vi "myRIO-1900 Customized FPGA.vi"() -> ()   [LabVIEW 2013]
doc: "This VI contains the NI myRIO FPGA shipping personality. This VI compiles and runs on the NI myRIO FPGA target. You can modify this VI to suit your application needs. National Instruments recommends that you only add new FPGA code to this VI and do not modify the existing code. This VI might not work correctly with the myRIO VIs if you modify the existing code."
uses:
  Sub VIs/Utilities/Start Boolean.ctl
  <vilib>/Platform/TimedLoop/XDataNode/timing_clust.ctl
  <vilib>/Platform/TimedLoop/XDataNode/nitl_modes.ctl
  <vilib>/Platform/TimedLoop/XDataNode/wakeup.ctl
  <vilib>/rvi/Emulation/niFpgaSctlEmulationGetInTimedLoop.vi
  <vilib>/rvi/Emulation/niFpgaEmulationReportErrorSimple.vi
  <vilib>/rvi/Emulation/niFpgaGetClockAttributes.vi
  <vilib>/rvi/Emulation/niFpgaCriticalErrorInLSC.vi
  <vilib>/rvi/interface/RandomDataEmulation/niFpgaRandomDataHandleErrors.vi
  <vilib>/rvi/interface/RandomDataEmulation/nirviRandomDataFPGAFIFO.vi
  <vilib>/rvi/eio/common/nirviEmuTemplateMethod_errors.vi
  <vilib>/rvi/eio/common/nirviEmuTemplatePropertyGet_noerrors.vi
  <vilib>/Platform/TimedLoop/XDataNode/XDataNode.xnode
  <vilib>/rvi/DataTransferAndStorage/Container/XNode/niFpgaContainer.xnode
  <vilib>/rvi/interface/RandomDataEmulation/nirviRandomDataFpgaReadWriteTemplate.vi
  <vilib>/eio/EIONode/EIONode.xnode
  <vilib>/eio/EIOPropertyNode/EIOPropertyNode.xnode
  <vilib>/Platform/TimedLoop/XDataNode/XDNodeRunTimeDep.lvlib
  <vilib>/rvi/eio/common/nirviEmuTemplatePropertyGet_errors.vi
  <vilib>/rvi/eio/common/nirviEmuTemplatePropertySet_errors.vi
  <vilib>/rvi/eio/common/nirviEmuTemplatePropertySet_noerrors.vi
panel:
  in  "LEDMatrix.clkdiv":u8(ring) items=["36 fps", "72 fps", "144 fps", "288 fps"]
  in  "LEDMatrix.origin":bool
  in  "LEDMatrix.Clear":bool
  in  "LEDMatrix.ClearColor":u32(colorbox)=16728810
  out "ACC.SCALE.WGHT":u16
  out "SYS.ACC_SCALE.RDY":bool
  out "AO.SYS.STAT":bool
  out "AI.B_1.WGHT":u32
  out "AO.B_0.WGHT":u32
  out "AO.B_1.WGHT":u32
  out "AO.B_0.OFST":u32
  out "AO.B_1.OFST":u32
  out "AO.A_0.WGHT":u32
  out "AO.A_1.WGHT":u32
  out "AO.C_0.WGHT":u32
  out "AO.C_1.WGHT":u32
  out "AO.AudioOut_L.WGHT":u32
  out "AO.AudioOut_R.WGHT":u32
  out "AO.A_0.OFST":u32
  out "AO.C_0.OFST":u32
  out "AO.C_1.OFST":u32
  out "AO.AudioOut_L.OFST":u32
  out "AO.AudioOut_R.OFST":u32
  out "AO.A_1.OFST":u32
  out "SYS.AO_SCALE.RDY":bool
  out "SYS.AI_SCALE.RDY":bool
  out "AI.A_1.OFST":u32
  out "AI.A_2.OFST":u32
  out "AI.A_3.OFST":u32
  out "AI.B_0.OFST":u32
  out "AI.B_1.OFST":u32
  out "AI.B_2.OFST":u32
  out "AI.B_3.OFST":u32
  out "AI.C_0.OFST":u32
  out "AI.C_1.OFST":u32
  out "AI.AudioIn_L.OFST":u32
  out "AI.AudioIn_R.OFST":u32
  out "AI.A_0.OFST":u32
  out "AI.AudioIn_R.WGHT":u32
  out "AI.AudioIn_L.WGHT":u32
  out "AI.C_1.WGHT":u32
  out "AI.C_0.WGHT":u32
  out "AI.B_3.WGHT":u32
  out "AI.B_2.WGHT":u32
  out "AI.B_0.WGHT":u32
  out "AI.A_3.WGHT":u32
  out "AI.A_2.WGHT":u32
  out "AI.A_1.WGHT":u32
  out "AI.A_0.WGHT":u32
  out "DI.BTN":u8 format="%08b"
  in  "DO.LED3:0":u8 format="%04b"
  out "ACC.Z.VAL":u16
  out "SYS.ACC.RDY":bool
  out "ACC.Y.VAL":u16
  out "ACC.X.VAL":u16
  in  "AO.SYS.GO":T1
  in  "AO.AudioOut_L.VAL":u16
  in  "AO.AudioOut_R.VAL":u16
  out "AI.AudioIn_L.VAL":u16
  out "AI.AudioIn_R.VAL":u16
  in  "DIO.B_15:8.OUT":u8 format="%08b"
  in  "DIO.B_15:8.DIR":u8 format="%08b"
  out "DIO.B_15:8.IN":u8 format="%08b"
  in  "DIO.A_15:8.DIR":u8 format="%08b"
  in  "DIO.A_15:8.OUT":u8 format="%08b"
  out "DIO.A_15:8.IN":u8 format="%08b"
  in  "PWM.C_0.MAX":u16
  in  "PWM.C_0.CMP":u16
  out "PWM.C_0.CNTR":u16
  in  "PWM.C_0.CNFG":u8 format="%08b"
  in  "PWM.C_0.CS":u8
  in  "PWM.C_1.MAX":u16
  in  "PWM.C_1.CMP":u16
  out "PWM.C_1.CNTR":u16
  in  "PWM.C_1.CNFG":u8 format="%08b"
  in  "PWM.C_1.CS":u8
  out "ENC.C_1.STAT":u8 format="%08b"
  out "ENC.C_1.CNTR":u32
  in  "ENC.C_1.CNFG":u8 format="%08b"
  out "ENC.C_0.STAT":u8 format="%08b"
  out "ENC.C_0.CNTR":u32
  in  "ENC.C_0.CNFG":u8 format="%08b"
  in  "SYS.SELECTA":u8 format="%08b"
  in  "SYS.SELECTC":u8 format="%08b"
  in  "SYS.SELECTB":u8 format="%08b"
  in  "AO.C_1.VAL":u16
  in  "AO.C_0.VAL":u16
  out "AI.C_0.VAL":u16
  out "AI.C_1.VAL":u16
  in  "DIO.C_7:0.OUT":u8 format="%08b"
  in  "DIO.C_7:0.DIR":u8 format="%08b"
  out "DIO.C_7:0.IN":u8 format="%08b"
  in  "DIO.A_7:0.DIR":u8 format="%08b"
  in  "DIO.A_7:0.OUT":u8 format="%08b"
  out "DIO.A_7:0.IN":u8 format="%08b"
  in  "PWM.B_0.CMP":u16
  in  "PWM.B_0.MAX":u16
  out "PWM.B_0.CNTR":u16
  in  "PWM.B_0.CNFG":u8 format="%08b"
  in  "PWM.B_0.CS":u8
  in  "PWM.B_1.CMP":u16
  in  "PWM.B_1.MAX":u16
  out "PWM.B_1.CNTR":u16
  in  "PWM.B_1.CNFG":u8 format="%08b"
  in  "PWM.B_1.CS":u8
  in  "PWM.B_2.CMP":u16
  in  "PWM.B_2.MAX":u16
  out "PWM.B_2.CNTR":u16
  in  "PWM.B_2.CNFG":u8 format="%08b"
  in  "PWM.B_2.CS":u8
  out "SYS.RDY":bool
  out "SYS.AI.RDY":bool
  in  "I2C.B.GO":T1
  in  "I2C.A.GO":T1
  in  "I2C.A.CNFG":u8 format="%08b"
  in  "I2C.B.CNFG":u8 format="%08b"
  in  "I2C.A.DATO":u8
  out "I2C.A.DATI":u8
  in  "I2C.A.ADDR":u8 format="%08b"
  in  "I2C.A.CNTR":u8
  in  "I2C.B.DATO":u8
  out "I2C.B.DATI":u8
  in  "I2C.B.ADDR":u8 format="%08.0f"
  in  "I2C.B.CNTR":u8
  in  "I2C.A.CNTL":u8 format="%08b"
  out "I2C.A.STAT":u8 format="%08b"
  in  "I2C.B.CNTL":u8 format="%08b"
  out "I2C.B.STAT":u8 format="%08b"
  out "SPI.A.STAT":u8 format="%08b"
  in  "SPI.A.GO":T1
  out "ENC.A.STAT":u8 format="%08b"
  out "ENC.A.CNTR":u32
  in  "ENC.A.CNFG":u8 format="%08b"
  in  "SPI.A.CNT":u16
  in  "SPI.A.CNFG":u16 format="%016b"
  out "SPI.A.DATI":u16
  in  "SPI.A.DATO":u16
  in  "PWM.A_0.MAX":u16
  in  "PWM.A_0.CMP":u16
  out "PWM.A_0.CNTR":u16
  in  "PWM.A_0.CNFG":u8 format="%08b"
  in  "PWM.A_0.CS":u8
  in  "PWM.A_1.CMP":u16
  in  "PWM.A_1.MAX":u16
  out "PWM.A_1.CNTR":u16
  in  "PWM.A_1.CNFG":u8 format="%08b"
  in  "PWM.A_1.CS":u8
  in  "PWM.A_2.CMP":u16
  in  "PWM.A_2.MAX":u16
  out "PWM.A_2.CNTR":u16
  in  "PWM.A_2.CNFG":u8 format="%08b"
  in  "PWM.A_2.CS":u8
  out "AI.A_0.VAL":u16
  out "AI.A_1.VAL":u16
  out "AI.A_2.VAL":u16
  out "AI.A_3.VAL":u16
  out "AI.B_0.VAL":u16
  out "AI.B_1.VAL":u16
  out "AI.B_2.VAL":u16
  out "AI.B_3.VAL":u16
  in  "AO.B_1.VAL":u16
  in  "AO.B_0.VAL":u16
  in  "AO.A_1.VAL":u16
  in  "AO.A_0.VAL":u16
  # "System"
  # "Onboard Devices"
  # "Connector A"
  # "Connector B"
  # "Connector C"
  # "Audio Connector"
  # "Accelerometer"
  # "Analog Input"
  # "Analog Output"
  # "Digital I/O"
  # "Counters / PWM"
  # "SPI Master"
  # "Analog Input"
  # "Analog Output"
  # "Digital I/O"
  # "Counters / PWM"
  # "SPI Master"
  # "Analog Input"
  # "Analog Output"
  # "Digital I/O"
  # "Counters / PWM"
  # "Analog Input"
  # "Encoders"
  # "Buttons & LEDs"
  # "I2C Master"
  # "I2C Master"
  # "Encoders"
  # "Encoders"
  # "Analog Output"
  # "IO Configuration"
  # "IO Configuration"
  # "IO Configuration"
  # "LED Matrix"
  # "Make LEDMatrix.origin TRUE whenever the first element from FIFO \nis to be at the top left of the LED Matrix. Must reset it to\nFALSE before setting to TRUE again."
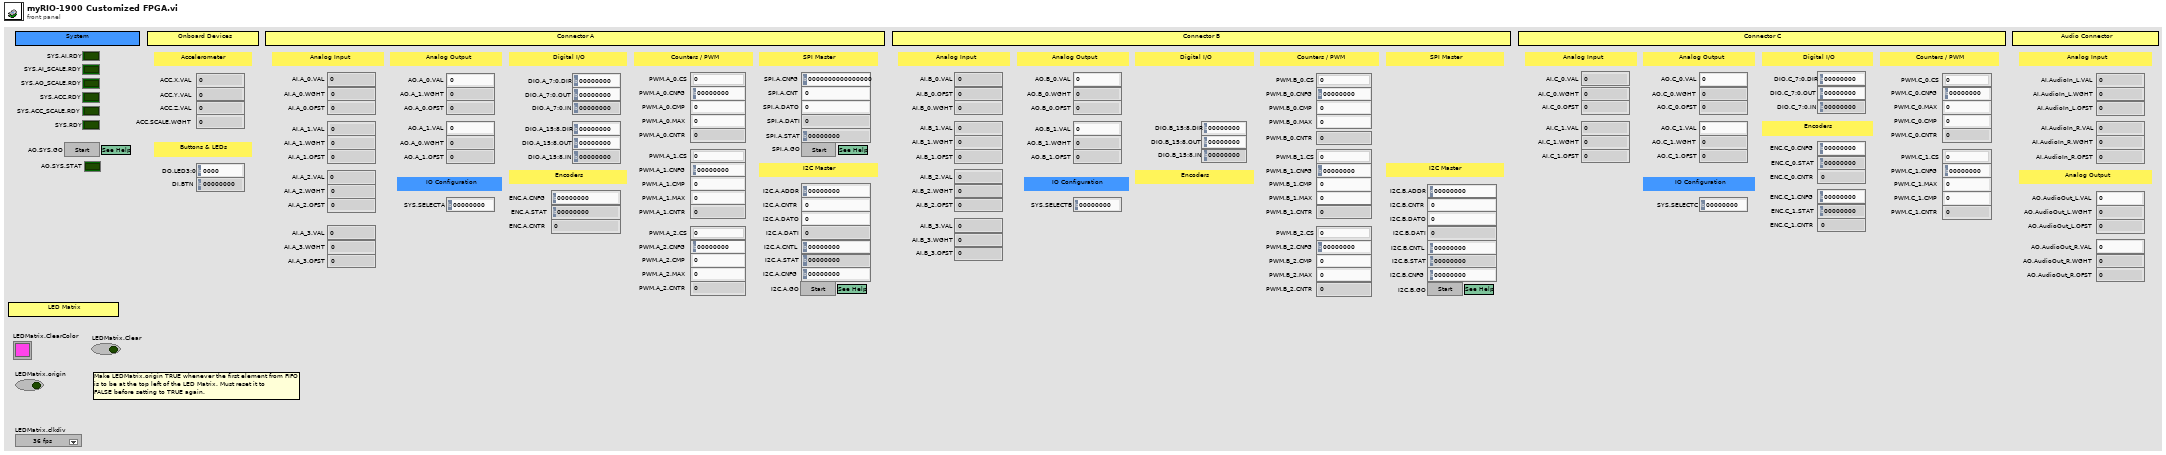
[diagram p1: front panel]
types:
  T1 = typedef "Start Boolean.ctl" = bool
  T2 = typedef "XDNodeRunTimeDep.lvlib/timing_clust.ctl" = cluster{"Expected End [f-1]":u64, "Actual End [f-1]":u64, "Finished Late? [f-1]":bool, "Expected End [i-1]":u64, "Actual End [i-1]":u64, "Finished Late? [i-1]":bool, "Expected Start [i]":u64, "Actual Start [i]":u64, "Expected Start [f]":u64, "Actual Start [f]":u64, "Source Name":string, "Structure Name":string, "Period":i64, "Deadline":i64, "Offset":i64, "Start":i64, "Priority":i32, "Timeout":i32, "Mode":T3, "Wakeup Reason":T4, "Error":errorcluster, "Source Type":string, "Secondary Source Type":string, "Global End Time":u64, "Global Start Time":u64, "Frame Duration":u64, "Iteration Duration":u64, "Assigned CPU":i32, "I/O Scan Engine Mode":u32}
  T3 = typedef "XDNodeRunTimeDep.lvlib/nitl_modes.ctl" = enum32{"No Change", "Process missed periods, maintain original phase", "Discard missed periods, maintain original phase", "Process missed periods, ignore original phase", "Discard missed periods, ignore original phase"}
  T4 = typedef "XDNodeRunTimeDep.lvlib/wakeup.ctl" = enum32{"Normal", "Aborted", "Asynchronous wakeup", "Timing source error", "Timed loop error", "Timeout"}
diagram:
  # "NOTE: The SYS.RDY boolean MUST exist and must become TRUE at some point otherwise the myRIO API will not function correctly."
  # "All DIO operations occur inside one single cycle timed loop (SCTL) since the IO is shared."
  # "The analog input scaling values are stored on the hardware. The RDY boolean should be checked before the values are used otherwise the analog input vlaues could be scaled incorrectly.\n\nAfter the first iteration of the while loop, all indicators have valid values."
  # "The analog output scaling values are stored on the hardware. The RDY boolean should be checked before the values are used otherwise the analog output vlaues could be scaled incorrectly.\n\nAfter the first iteration of the while loop, all indicators have valid values."
  # "The accelerometer nodes takes some time before the values can first be read (this is due to the time taken to read from the acceleromter). An iteration of the while loop will not complete until the accelerometer values have been read.\n\nAfter the first iteration of the while loop, all indicators have valid values."
  # "The onboard accelerometer has a range of +/- 8g which translates to 256 bits/g. The scaling weight is hardcoded in the FPGA to allow for future updates with minimal changes in the myRIO code. The RDY boolean should be checked before the values are used otherwise the analog output vlaues could be scaled incorrectly.\n\nAfter the first iteration of the while loop, all indicators have valid values."
  # "Onboard Accelerometer Scaling"
  # "Analog Output Scaling Constants"
  # "Analog Input Scaling Constants"
  # "Onboard Accelerometer"
  # "Onboard DIO"
  # "Connector B DIO"
  # "There is some delay between when the FPGA code starts and the analog inputs, accelerometer, and scaling values outputs are valid. If the host wants to ensure that there are valid values in theses registers it should wait for each subsystem to finish its initialization process. \n\nWhen all subsystems have finished initializinig, the SYS.RDY indicator will be true, which can be polled by the host to determine the status of the FPGA. Alternatively, the host can poll the individual SYS.xx.RDY indicators to determine the status of the individual subsystems.\n\nThis loop continues indefinitely, essentially making SYS.RDY a read-only register."
  # "The analog input nodes takes some time before the values can first be read (this is due to the time taken to setup the ADC and convert the first reading). An iteration of the while loop will not complete until all the analog input channels have been sampled.\n\nAfter the first iteration of the while loop, all indicators have valid values."
  # "Note: On some hardware a \"ghosting effect\" may occur on any unconnected AI channels. For example, if channel AI0 is connected and channels AI1 - AI7 are not connected the the value read at AI0 may be seen on indicators AI1 - AI7. This is common for hardware that use a multiplexed (MUXed) Analog-to-Digital converter (ADC) since the input analog signal is used to charge a capacitor which does not discharge before the unconnected channel is read.\n\n\"Ghosting\" effect can be hidden be using an mask register which will be used to decide when the indicator should be updated."
  # "The analog output nodes take some time before values are written to the pins. The GO and STAT registers are used to handshake between the FPGA and host. When the host wants the values to be written it sets the GO register to true. If the host reads the STAT register before setting GO, it can then wait for the STAT register value to invert which will tell the host that the output values have been written."
  # "Connector A DIO"
  # "Connector C  DIO"
  # "Host Synchronization"
  # "Analog Output"
  # "Analog Input"
  n1 = while {
    stop <- FALSE stop-if-true
    n2 = local read "SYS.ACC_SCALE.RDY"() -> (w12:bool)
    n3 = local read "SYS.AO_SCALE.RDY"() -> (w13:bool)
    n4 = local read "SYS.AI_SCALE.RDY"() -> (w14:bool)
    n5 = local read "SYS.ACC.RDY"() -> (w15:bool)
    n6 = local read "SYS.AI.RDY"() -> (w17:bool)
    n7 = Compound Arithmetic op=AND(w17, w15, w14, w13, w12) -> (→"SYS.RDY":bool)
  }
  n8 = node-c288() -> (w2:T2)  [unwired: 1 in]
  n9 = while {
    i -> [w29]
    stop <- FALSE stop-if-true
    n10 = xnode "FPGA I/O Node"() -> ("ConnectorA/AI0"=→"AI.A_0.VAL":u16, "ConnectorA/AI1"=→"AI.A_1.VAL":u16, "ConnectorA/AI2"=→"AI.A_2.VAL":u16, "ConnectorA/AI3"=→"AI.A_3.VAL":u16, "ConnectorB/AI0"=→"AI.B_0.VAL":u16, "ConnectorB/AI1"=→"AI.B_1.VAL":u16, "ConnectorB/AI2"=→"AI.B_2.VAL":u16, "ConnectorB/AI3"=→"AI.B_3.VAL":u16, "ConnectorC/AI0"=w23:i16, "ConnectorC/AI1"=w22:i16, "AudioIn/Left"=w21:i16, "AudioIn/Right"=w20:i16)  [unwired: 12 in, 12 out]
    n11 = Greater Than 0?(x=w29) -> (x > 0?=→"SYS.AI.RDY":bool)
    n12 = To Unsigned Word Integer(number=w23) -> (unsigned 16bit integer=→"AI.C_0.VAL":u16)
    n13 = To Unsigned Word Integer(number=w22) -> (unsigned 16bit integer=→"AI.C_1.VAL":u16)
    n14 = To Unsigned Word Integer(number=w21) -> (unsigned 16bit integer=→"AI.AudioIn_L.VAL":u16)
    n15 = To Unsigned Word Integer(number=w20) -> (unsigned 16bit integer=→"AI.AudioIn_R.VAL":u16)
  }
  n16 = timed-loop {
    timing: w2 -> [_]
    timing-out: [_] -> w1
    stop <- FALSE stop-if-true
    # "For Debug"
    # "Make LEDMatrix.origin TRUE whenever the first element from FIFO \nis to be at the top left of the LED Matrix. Must reset it to\nFALSE before setting to TRUE again."
    n17 = xnode ("FIFO Method Node")("Timeout"=0) -> ("Element"=w46:u32, "Timed Out?"=w41:bool)  [unwired: 1 in, 1 out]
    n18 = Not(x=w41) -> (.not. x?=w42:bool)
    n19 = Select(t="LEDMatrix.ClearColor", s="LEDMatrix.Clear", f=w46) -> (s? t:f=w47:u32)
    n20 = Select(t=TRUE, s="LEDMatrix.Clear", f=w42) -> (s? t:f=w43:bool)
    n21 = xnode "FPGA I/O Node"("Component-Level IP\\origin"="LEDMatrix.origin") -> ()  [unwired: 1 in, 1 out]
    n22 = xnode "FPGA I/O Node"("Component-Level IP\\data_in32"=w47) -> ()  [unwired: 1 in, 1 out]
    n23 = xnode "FPGA I/O Node"("Component-Level IP\\data_valid"=w43) -> ()  [unwired: 1 in, 1 out]
    n24 = xnode "FPGA I/O Node"("Component-Level IP\\div"="LEDMatrix.clkdiv") -> ()  [unwired: 1 in, 1 out]
    n25 = xnode "FPGA I/O Node"() -> ("Component-Level IP\\frame"=w38:bool)  [unwired: 1 in, 1 out]
    n26 = xnode "FPGA I/O Node"() -> ("Component-Level IP\\clk_out"=w60:bool, "Component-Level IP\\r1"=w59:bool, "Component-Level IP\\r2"=w58:bool, "Component-Level IP\\b1"=w57:bool, "Component-Level IP\\b2"=w56:bool, "Component-Level IP\\g1"=w55:bool, "Component-Level IP\\g2"=w54:bool, "Component-Level IP\\a"=w53:bool, "Component-Level IP\\b"=w52:bool, "Component-Level IP\\c"=w51:bool, "Component-Level IP\\lat"=w50:bool, "Component-Level IP\\oe_n"=w49:bool)  [unwired: 12 in, 12 out]
    n27 = xnode "FPGA I/O Node"("ConnectorB/DIO5"=w53, "ConnectorB/DIO12"=w52, "ConnectorB/DIO6"=w51, "ConnectorB/DIO13"=w50, "ConnectorB/DIO8"=w49) -> ()  [unwired: 5 in, 5 out]
    n28 = xnode "FPGA I/O Node"("ConnectorB/DIO7"=w60, "ConnectorB/DIO0"=w59, "ConnectorB/DIO3"=w58, "ConnectorB/DIO2"=w57, "ConnectorB/DIO4"=w56, "ConnectorB/DIO1"=w55, "ConnectorB/DIO11"=w54) -> ()  [unwired: 7 in, 7 out]
    n29 = xnode "FPGA I/O Node"("ConnectorA/DIO0"=w38) -> ()  [unwired: 1 in, 1 out]
  }
  n30 = while {
    i -> [w66]
    stop <- FALSE stop-if-true
    n31 = Greater Than 0?(x=w66) -> (x > 0?=→"SYS.AI_SCALE.RDY":bool)
    n32 = xnode "FPGA I/O Property Node"("FPGA I/O In"=refnum<k21> "ConnectorA/AI0" ("FPGA I/O")) -> ("LSB Weight"=→"AI.A_0.WGHT":u32, "Offset"=w91:i32)  [unwired: 1 out]
    n33 = xnode "FPGA I/O Property Node"("FPGA I/O In"=refnum<k21> "ConnectorA/AI1" ("FPGA I/O")) -> ("LSB Weight"=→"AI.A_1.WGHT":u32, "Offset"=w79:i32)  [unwired: 1 out]
    n34 = xnode "FPGA I/O Property Node"("FPGA I/O In"=refnum<k21> "ConnectorA/AI2" ("FPGA I/O")) -> ("LSB Weight"=→"AI.A_2.WGHT":u32, "Offset"=w88:i32)  [unwired: 1 out]
    n35 = xnode "FPGA I/O Property Node"("FPGA I/O In"=refnum<k21> "ConnectorA/AI3" ("FPGA I/O")) -> ("LSB Weight"=→"AI.A_3.WGHT":u32, "Offset"=w87:i32)  [unwired: 1 out]
    n36 = xnode "FPGA I/O Property Node"("FPGA I/O In"=refnum<k21> "ConnectorB/AI0" ("FPGA I/O")) -> ("LSB Weight"=→"AI.B_0.WGHT":u32, "Offset"=w86:i32)  [unwired: 1 out]
    n37 = xnode "FPGA I/O Property Node"("FPGA I/O In"=refnum<k21> "ConnectorB/AI1" ("FPGA I/O")) -> ("LSB Weight"=→"AI.B_1.WGHT":u32, "Offset"=w85:i32)  [unwired: 1 out]
    n38 = xnode "FPGA I/O Property Node"("FPGA I/O In"=refnum<k21> "ConnectorB/AI2" ("FPGA I/O")) -> ("LSB Weight"=→"AI.B_2.WGHT":u32, "Offset"=w84:i32)  [unwired: 1 out]
    n39 = xnode "FPGA I/O Property Node"("FPGA I/O In"=refnum<k21> "ConnectorB/AI3" ("FPGA I/O")) -> ("LSB Weight"=→"AI.B_3.WGHT":u32, "Offset"=w83:i32)  [unwired: 1 out]
    n40 = xnode "FPGA I/O Property Node"("FPGA I/O In"=refnum<k21> "ConnectorC/AI0" ("FPGA I/O")) -> ("LSB Weight"=→"AI.C_0.WGHT":u32, "Offset"=w82:i32)  [unwired: 1 out]
    n41 = xnode "FPGA I/O Property Node"("FPGA I/O In"=refnum<k21> "ConnectorC/AI1" ("FPGA I/O")) -> ("LSB Weight"=→"AI.C_1.WGHT":u32, "Offset"=w81:i32)  [unwired: 1 out]
    n42 = xnode "FPGA I/O Property Node"("FPGA I/O In"=refnum<k21> "AudioIn/Left" ("FPGA I/O")) -> ("LSB Weight"=→"AI.AudioIn_L.WGHT":u32, "Offset"=w80:i32)  [unwired: 1 out]
    n43 = xnode "FPGA I/O Property Node"("FPGA I/O In"=refnum<k21> "AudioIn/Right" ("FPGA I/O")) -> ("LSB Weight"=→"AI.AudioIn_R.WGHT":u32, "Offset"=w90:i32)  [unwired: 1 out]
    n44 = To Unsigned Long Integer(number=w91) -> (unsigned 32bit integer=→"AI.A_0.OFST":u32)
    n45 = To Unsigned Long Integer(number=w79) -> (unsigned 32bit integer=→"AI.A_1.OFST":u32)
    n46 = To Unsigned Long Integer(number=w88) -> (unsigned 32bit integer=→"AI.A_2.OFST":u32)
    n47 = To Unsigned Long Integer(number=w87) -> (unsigned 32bit integer=→"AI.A_3.OFST":u32)
    n48 = To Unsigned Long Integer(number=w86) -> (unsigned 32bit integer=→"AI.B_0.OFST":u32)
    n49 = To Unsigned Long Integer(number=w85) -> (unsigned 32bit integer=→"AI.B_1.OFST":u32)
    n50 = To Unsigned Long Integer(number=w84) -> (unsigned 32bit integer=→"AI.B_2.OFST":u32)
    n51 = To Unsigned Long Integer(number=w83) -> (unsigned 32bit integer=→"AI.B_3.OFST":u32)
    n52 = To Unsigned Long Integer(number=w82) -> (unsigned 32bit integer=→"AI.C_0.OFST":u32)
    n53 = To Unsigned Long Integer(number=w81) -> (unsigned 32bit integer=→"AI.C_1.OFST":u32)
    n54 = To Unsigned Long Integer(number=w80) -> (unsigned 32bit integer=→"AI.AudioIn_L.OFST":u32)
    n55 = To Unsigned Long Integer(number=w90) -> (unsigned 32bit integer=→"AI.AudioIn_R.OFST":u32)
  }
  n56 = while {
    stop <- FALSE stop-if-true
    n57 = feedback #1(FALSE) -> (w117:bool)
    n58 = case shown="True" "AO.SYS.GO" {
      tunnel: "AO.C_0.VAL" -> [_ w139]
      tunnel: "AO.C_1.VAL" -> [_ w138]
      tunnel: "AO.A_0.VAL" -> [_ w143]
      tunnel: "AO.A_1.VAL" -> [_ w142]
      tunnel: "AO.B_0.VAL" -> [_ w141]
      tunnel: "AO.B_1.VAL" -> [_ w140]
      tunnel: "AO.AudioOut_L.VAL" -> [_ w135]
      tunnel: "AO.AudioOut_R.VAL" -> [_ w134]
      tunnel: w117 -> [w128 w131]
      tunnel: [w128 w129] -> w115
      frame False {
      }
      frame True {
        n59 = To Word Integer(number=w139) -> (16bit integer=w137:i16)
        n60 = To Word Integer(number=w138) -> (16bit integer=w136:i16)
        n61 = To Word Integer(number=w135) -> (16bit integer=w133:i16)
        n62 = To Word Integer(number=w134) -> (16bit integer=w132:i16)
        n63 = flat-sequence {
          tunnel: w143 -> [w152]
          tunnel: w142 -> [w151]
          tunnel: w141 -> [w150]
          tunnel: w140 -> [w149]
          tunnel: w137 -> [w148]
          tunnel: w136 -> [w147]
          tunnel: w133 -> [w146]
          tunnel: w132 -> [w145]
          tunnel: w131 -> [w144]
          tunnel: [w144] -> w130
          tunnel: w130 -> [w154]
          tunnel: [w153] -> w129
          frame #0 {
            n64 = xnode "FPGA I/O Node"("ConnectorA/AO0"=w152, "ConnectorA/AO1"=w151, "ConnectorB/AO0"=w150, "ConnectorB/AO1"=w149, "ConnectorC/AO0"=w148, "ConnectorC/AO1"=w147, "AudioOut/Left"=w146, "AudioOut/Right"=w145) -> ()  [unwired: 8 in, 8 out]
          }
          frame #1 {
            n65 = Not(x=w154) -> (.not. x?=w153:bool)
          }
        }
      }
    }
    "AO.SYS.STAT" <- w115
    n66 = feedback-in #1(w115) -> ()
  }
  n67 = node-c288(w1) -> ()
  n68 = while {
    i -> [w176]
    stop <- FALSE stop-if-true
    n69 = Greater Than 0?(x=w176) -> (x > 0?=→"SYS.AO_SCALE.RDY":bool)
    n70 = xnode "FPGA I/O Property Node"("FPGA I/O In"=refnum<k21> "ConnectorA/AO0" ("FPGA I/O")) -> ("LSB Weight"=→"AO.A_0.WGHT":u32, "Offset"=w187:i32)  [unwired: 1 out]
    n71 = xnode "FPGA I/O Property Node"("FPGA I/O In"=refnum<k21> "ConnectorA/AO1" ("FPGA I/O")) -> ("LSB Weight"=→"AO.A_1.WGHT":u32, "Offset"=w179:i32)  [unwired: 1 out]
    n72 = xnode "FPGA I/O Property Node"("FPGA I/O In"=refnum<k21> "ConnectorB/AO0" ("FPGA I/O")) -> ("LSB Weight"=→"AO.B_0.WGHT":u32, "Offset"=w185:i32)  [unwired: 1 out]
    n73 = xnode "FPGA I/O Property Node"("FPGA I/O In"=refnum<k21> "ConnectorB/AO1" ("FPGA I/O")) -> ("LSB Weight"=→"AO.B_1.WGHT":u32, "Offset"=w184:i32)  [unwired: 1 out]
    n74 = xnode "FPGA I/O Property Node"("FPGA I/O In"=refnum<k21> "ConnectorC/AO0" ("FPGA I/O")) -> ("LSB Weight"=→"AO.C_0.WGHT":u32, "Offset"=w183:i32)  [unwired: 1 out]
    n75 = xnode "FPGA I/O Property Node"("FPGA I/O In"=refnum<k21> "ConnectorC/AO1" ("FPGA I/O")) -> ("LSB Weight"=→"AO.C_1.WGHT":u32, "Offset"=w182:i32)  [unwired: 1 out]
    n76 = xnode "FPGA I/O Property Node"("FPGA I/O In"=refnum<k21> "AudioOut/Left" ("FPGA I/O")) -> ("LSB Weight"=→"AO.AudioOut_L.WGHT":u32, "Offset"=w181:i32)  [unwired: 1 out]
    n77 = xnode "FPGA I/O Property Node"("FPGA I/O In"=refnum<k21> "AudioOut/Right" ("FPGA I/O")) -> ("LSB Weight"=→"AO.AudioOut_R.WGHT":u32, "Offset"=w180:i32)  [unwired: 1 out]
    n78 = To Unsigned Long Integer(number=w187) -> (unsigned 32bit integer=→"AO.A_0.OFST":u32)
    n79 = To Unsigned Long Integer(number=w179) -> (unsigned 32bit integer=→"AO.A_1.OFST":u32)
    n80 = To Unsigned Long Integer(number=w185) -> (unsigned 32bit integer=→"AO.B_0.OFST":u32)
    n81 = To Unsigned Long Integer(number=w184) -> (unsigned 32bit integer=→"AO.B_1.OFST":u32)
    n82 = To Unsigned Long Integer(number=w183) -> (unsigned 32bit integer=→"AO.C_0.OFST":u32)
    n83 = To Unsigned Long Integer(number=w182) -> (unsigned 32bit integer=→"AO.C_1.OFST":u32)
    n84 = To Unsigned Long Integer(number=w181) -> (unsigned 32bit integer=→"AO.AudioOut_L.OFST":u32)
    n85 = To Unsigned Long Integer(number=w180) -> (unsigned 32bit integer=→"AO.AudioOut_R.OFST":u32)
  }
  n86 = node-c288() -> (w4:T2)  [unwired: 1 in]
  n87 = timed-loop {
    timing: w4 -> [_]
    timing-out: [_] -> w3
    stop <- _ stop-if-true
    n88 = xnode "FPGA I/O Node"() -> ("Button0"=w198:bool)  [unwired: 1 in, 1 out]
    n89 = Number To Boolean Array(number="DO.LED3:0") -> (Boolean array=w194:bool[])
    n90 = Build Array(w198) -> (w197:bool[])
    n91 = Index Array(array=w194) -> (element #1=w193:bool, element #2=w192:bool, element #3=w191:bool, element #4=w190:bool)  [unwired: 4 in]
    n92 = Boolean Array To Number(Boolean array=w197) -> (number=→"DI.BTN":u8)
    n93 = xnode "FPGA I/O Node"("LED0"=w193, "LED1"=w192, "LED2"=w191, "LED3"=w190) -> ()  [unwired: 4 in, 4 out]
  }
  n94 = while {
    i -> [w205]
    stop <- FALSE stop-if-true
    n95 = xnode "FPGA I/O Node"() -> ("AccelerationX"=w208:i16, "AccelerationY"=w207:i16, "AccelerationZ"=w206:i16)  [unwired: 3 in, 3 out]
    n96 = Greater Than 0?(x=w205) -> (x > 0?=→"SYS.ACC.RDY":bool)
    n97 = To Unsigned Word Integer(number=w208) -> (unsigned 16bit integer=→"ACC.X.VAL":u16)
    n98 = To Unsigned Word Integer(number=w207) -> (unsigned 16bit integer=→"ACC.Y.VAL":u16)
    n99 = To Unsigned Word Integer(number=w206) -> (unsigned 16bit integer=→"ACC.Z.VAL":u16)
  }
  n100 = while {
    i -> [w212]
    stop <- FALSE stop-if-true
    # "The onboard accelerometer has a range of +/-8g which translates to 256 bits / g. The scaling weight is hardcoded in the FPGA to"
    n101 = Greater Than 0?(x=w212) -> (x > 0?=→"SYS.ACC_SCALE.RDY":bool)
    "ACC.SCALE.WGHT" <- u16 256 ("ACC.SCALE.WGHT")
  }
  n102 = node-c288(w3) -> ()
  n103 = node-c288() -> (w8:T2)  [unwired: 1 in]
  n104 = timed-loop {
    timing: w8 -> [_]
    timing-out: [_] -> w7
    stop <- _ stop-if-true
    # "DIO / Encoder"
    # "DIO / I2C Master"
    # "DIO / PWM"
    # "DIO"
    # "DIO"
    # "DIO/ SPI Master"
    n105 = call "Split HDC Bank1 DIO.vi"("IN 7:0"="DIO.A_7:0.OUT") -> ("OUT 3:0"=w301:fxp<+,4,4>, "OUT 4"=w214:bool, "OUT 7:5"=w298:fxp<+,3,3>)
    n106 = call "Split HDC Bank1 DIO.vi"("IN 7:0"="DIO.A_7:0.DIR") -> ("OUT 3:0"=w300:fxp<+,4,4>, "OUT 4"=w299:bool, "OUT 7:5"=w297:fxp<+,3,3>)
    n107 = call "Split HDC Function Select.vi"("IN 7:0"="SYS.SELECTA") -> ("OUT 1:0"=w235:fxp<+,2,2>, "OUT 7"=w230:bool, "OUT 2"=w234:bool, "OUT 3"=w233:bool, "OUT 4"=w232:bool, "OUT 5"=w231:bool)
    n108 = call "DIO 4-bit.vi"("DIO0 Refnum"=refnum<k21> "ConnectorA/DIO0", "DIO1 Refnum"=refnum<k21> "ConnectorA/DIO1", "DIO2 Refnum"=refnum<k21> "ConnectorA/DIO2", "DIR 3:0"=w300, "OUT 3:0"=w301, "DIO3 Refnum"=refnum<k21> "ConnectorA/DIO3") -> ("IN 3:0"=w272:fxp<+,4,4>)  [unwired: 5 in]
    n109 = call "DIO 1-bit.vi"("DIR"=w299, "OUT"=w214, "DIO Refnum"=refnum<k21> "ConnectorA/DIO4") -> ("IN"=w271:bool)  [unwired: 8 in]
    n110 = call "DIO_SPI.vi"("DIO.2:0.OUT"=w298, "DIO.2:0.DIR"=w297, "SPI.CNT"="SPI.A.CNT", "SPI.CNFG"="SPI.A.CNFG", "SPI.DATO"="SPI.A.DATO", "SPI.GO"="SPI.A.GO", "DIO.2/SPI.MOSI Refnum"=refnum<k21> "ConnectorA/DIO7" ("DIO.2/SPI.SCLK"), "SELECT.1:0"=w235, "DIO.1/SPI.MISO Refnum"=refnum<k21> "ConnectorA/DIO6" ("DIO.1/SPI.MOSI"), "DIO.0/SPI.SCLK Refnum"=refnum<k21> "ConnectorA/DIO5" ("DIO.0/SPI.MISO")) -> ("DIO.2:0.IN"=w270:fxp<+,3,3>, "SPI.DATI"=→"SPI.A.DATI":u16, "SPI.STAT"=→"SPI.A.STAT":u8)  [unwired: 7 in]
    n111 = call "Join HDC Bank1 DIO.vi"("IN 7:5"=w270, "IN 4"=w271, "IN 3:0"=w272) -> ("OUT 7:0"=→"DIO.A_7:0.IN":u8)
    n112 = call "Split HDC Bank2 DIO.vi"("IN 7:0"="DIO.A_15:8.OUT") -> ("OUT 5"=w216:bool, "OUT 7:6"=w240:fxp<+,2,2>, "OUT 4:3"=w218:fxp<+,2,2>, "OUT 2"=w220:bool, "OUT 0"=w224:bool, "OUT 1"=w223:bool)  [unwired: 2 in]
    n113 = call "Split HDC Bank2 DIO.vi"("IN 7:0"="DIO.A_15:8.DIR") -> ("OUT 5"=w215:bool, "OUT 7:6"=w239:fxp<+,2,2>, "OUT 4:3"=w217:fxp<+,2,2>, "OUT 2"=w219:bool, "OUT 0"=w222:bool, "OUT 1"=w221:bool)  [unwired: 2 in]
    n114 = call "DIO_PWM.vi"("DIO.OUT"=w224, "DIO.DIR"=w222, "PWM.CS"="PWM.A_0.CS", "PWM.CNFG"="PWM.A_0.CNFG", "PWM.CMP"="PWM.A_0.CMP", "PWM.MAX"="PWM.A_0.MAX", "DIO/PWM"=refnum<k21> "ConnectorA/DIO8", "SELECT"=w234) -> ("DIO.IN"=w229:bool, "PWM.CNTR"=→"PWM.A_0.CNTR":u16)  [unwired: 10 in]
    n115 = call "DIO_PWM.vi"("DIO.OUT"=w223, "DIO.DIR"=w221, "PWM.CS"="PWM.A_1.CS", "PWM.CNFG"="PWM.A_1.CNFG", "PWM.CMP"="PWM.A_1.CMP", "PWM.MAX"="PWM.A_1.MAX", "DIO/PWM"=refnum<k21> "ConnectorA/DIO9", "SELECT"=w233) -> ("DIO.IN"=w228:bool, "PWM.CNTR"=→"PWM.A_1.CNTR":u16)  [unwired: 10 in]
    n116 = call "DIO_PWM.vi"("DIO.OUT"=w220, "DIO.DIR"=w219, "PWM.CS"="PWM.A_2.CS", "PWM.CNFG"="PWM.A_2.CNFG", "PWM.CMP"="PWM.A_2.CMP", "PWM.MAX"="PWM.A_2.MAX", "DIO/PWM"=refnum<k21> "ConnectorA/DIO10", "SELECT"=w232) -> ("DIO.IN"=w227:bool, "PWM.CNTR"=→"PWM.A_2.CNTR":u16)  [unwired: 10 in]
    n117 = call "DIO_Encoder.vi"("DIO.1:0.OUT"=w218, "DIO.1:0.DIR"=w217, "QE.CNFG"="ENC.A.CNFG", "DIO.1/QE.B"=refnum<k21> "ConnectorA/DIO12", "SELECT"=w231, "DIO.0/QE.A"=refnum<k21> "ConnectorA/DIO11") -> ("DIO.1:0.IN"=w226:fxp<+,2,2>, "QE.CNTR"=→"ENC.A.CNTR":u32, "QE.STAT"=→"ENC.A.STAT":u8)  [unwired: 11 in]
    n118 = call "DIO 1-bit.vi"("DIR"=w215, "OUT"=w216, "DIO Refnum"=refnum<k21> "ConnectorA/DIO13") -> ("IN"=w225:bool)  [unwired: 8 in]
    n119 = call "DIO_I2C.vi"("DIO.1:0.OUT"=w240, "DIO.1:0.DIR"=w239, "I2C.CNFG"="I2C.A.CNFG", "I2C.CNTL"="I2C.A.CNTL", "I2C.ADDR"="I2C.A.ADDR", "I2C.DATO"="I2C.A.DATO", "DIO.1/I2C.SDA"=refnum<k21> "ConnectorA/DIO15" ("DIO.1/I2C.SCL"), "I2C.CNTR"="I2C.A.CNTR", "DIO.0/I2C.SCL"=refnum<k21> "ConnectorA/DIO14" ("DIO.0/I2C.SDA"), "Execute?"="I2C.A.GO", "SELECT"=w230) -> ("DIO.1:0.IN"=w237:fxp<+,2,2>, "I2C.DATI"=→"I2C.A.DATI":u8, "I2C.STAT"=→"I2C.A.STAT":u8)  [unwired: 6 in]
    n120 = call "Join HDC Bank2 DIO.vi"("IN 7:6"=w237, "IN 5"=w225, "IN 4:3"=w226, "IN 0"=w229, "IN 2"=w227, "IN 1"=w228) -> ("OUT 7:0"=→"DIO.A_15:8.IN":u8)  [unwired: 4 in]
  }
  n121 = node-c288(w7) -> ()
  n122 = node-c288() -> (w6:T2)  [unwired: 1 in]
  n123 = timed-loop {
    timing: w6 -> [_]
    timing-out: [_] -> w5
    stop <- _ stop-if-true
    # "DIO / I2C Master"
    # "DIO / PWM"
    # "DIO"
    n124 = call "Split HDC Function Select.vi"("IN 7:0"="SYS.SELECTB") -> ("OUT 7"=w342:bool, "OUT 2"=w345:bool, "OUT 3"=w344:bool, "OUT 4"=w343:bool)  [unwired: 2 out]
    n125 = call "Split HDC Bank2 DIO.vi"("IN 7:0"="DIO.B_15:8.OUT") -> ("OUT 7:6"=w348:fxp<+,2,2>, "OUT 2"=w312:bool, "OUT 0"=w314:bool, "OUT 1"=w313:bool)  [unwired: 2 in, 2 out]
    n126 = call "Split HDC Bank2 DIO.vi"("IN 7:0"="DIO.B_15:8.DIR") -> ("OUT 7:6"=w347:fxp<+,2,2>, "OUT 2"=w309:bool, "OUT 0"=w311:bool, "OUT 1"=w310:bool)  [unwired: 2 in, 2 out]
    n127 = call "DIO_PWM.vi"("DIO.OUT"=w314, "DIO.DIR"=w311, "PWM.CS"="PWM.B_0.CS", "PWM.CNFG"="PWM.B_0.CNFG", "PWM.CMP"="PWM.B_0.CMP", "PWM.MAX"="PWM.B_0.MAX", "DIO/PWM"=refnum<k21> "ConnectorB/DIO8", "SELECT"=w345) -> ("DIO.IN"=w308:bool, "PWM.CNTR"=→"PWM.B_0.CNTR":u16)  [unwired: 10 in]
    n128 = call "DIO_PWM.vi"("DIO.OUT"=w313, "DIO.DIR"=w310, "PWM.CS"="PWM.B_1.CS", "PWM.CNFG"="PWM.B_1.CNFG", "PWM.CMP"="PWM.B_1.CMP", "PWM.MAX"="PWM.B_1.MAX", "DIO/PWM"=refnum<k21> "ConnectorB/DIO9", "SELECT"=w344) -> ("DIO.IN"=w307:bool, "PWM.CNTR"=→"PWM.B_1.CNTR":u16)  [unwired: 10 in]
    n129 = call "DIO_PWM.vi"("DIO.OUT"=w312, "DIO.DIR"=w309, "PWM.CS"="PWM.B_2.CS", "PWM.CNFG"="PWM.B_2.CNFG", "PWM.CMP"="PWM.B_2.CMP", "PWM.MAX"="PWM.B_2.MAX", "DIO/PWM"=refnum<k21> "ConnectorB/DIO10", "SELECT"=w343) -> ("DIO.IN"=w306:bool, "PWM.CNTR"=→"PWM.B_2.CNTR":u16)  [unwired: 10 in]
    n130 = call "DIO_I2C.vi"("DIO.1:0.OUT"=w348, "DIO.1:0.DIR"=w347, "I2C.CNFG"="I2C.B.CNFG", "I2C.CNTL"="I2C.B.CNTL", "I2C.ADDR"="I2C.B.ADDR", "I2C.DATO"="I2C.B.DATO", "DIO.1/I2C.SDA"=refnum<k21> "ConnectorB/DIO15" ("DIO.1/I2C.SCL"), "I2C.CNTR"="I2C.B.CNTR", "DIO.0/I2C.SCL"=refnum<k21> "ConnectorB/DIO14" ("DIO.0/I2C.SDA"), "Execute?"="I2C.B.GO", "SELECT"=w342) -> ("DIO.1:0.IN"=w346:fxp<+,2,2>, "I2C.DATI"=→"I2C.B.DATI":u8, "I2C.STAT"=→"I2C.B.STAT":u8)  [unwired: 6 in]
    n131 = call "Join HDC Bank2 DIO.vi"("IN 7:6"=w346, "IN 5"=FALSE, "IN 4:3"=fxp<+,2,2> 0.0, "IN 0"=w308, "IN 2"=w306, "IN 1"=w307) -> ("OUT 7:0"=→"DIO.B_15:8.IN":u8)  [unwired: 4 in]
  }
  n132 = node-c288(w5) -> ()
  n133 = node-c288() -> (w10:T2)  [unwired: 1 in]
  n134 = timed-loop {
    timing: w10 -> [_]
    timing-out: [_] -> w9
    stop <- _ stop-if-true
    n135 = call "Split myDAQ DIO.vi"("IN 7:0"="DIO.C_7:0.OUT") -> ("OUT 2, OUT0"=w374:fxp<+,2,2>, "OUT 1"=w373:bool, "OUT 3"=w372:bool, "OUT 7"=w369:bool, "OUT 6, OUT 4"=w371:fxp<+,2,2>, "OUT 5"=w370:bool)  [unwired: 4 in]
    n136 = call "Split myDAQ DIO.vi"("IN 7:0"="DIO.C_7:0.DIR") -> ("OUT 2, OUT0"=w368:fxp<+,2,2>, "OUT 1"=w367:bool, "OUT 3"=w366:bool, "OUT 7"=w363:bool, "OUT 6, OUT 4"=w365:fxp<+,2,2>, "OUT 5"=w364:bool)  [unwired: 4 in]
    n137 = call "Split myDAQ Function Select.vi"("IN 7:0"="SYS.SELECTC") -> ("OUT 0"=w380:bool, "OUT 1"=w379:bool, "OUT 2"=w378:bool, "OUT 3"=w377:bool)  [unwired: 2 in]
    n138 = call "DIO_Encoder.vi"("DIO.1:0.OUT"=w374, "DIO.1:0.DIR"=w368, "QE.CNFG"="ENC.C_0.CNFG", "DIO.1/QE.B"=refnum<k21> "ConnectorC/DIO2", "SELECT"=w380, "DIO.0/QE.A"=refnum<k21> "ConnectorC/DIO0") -> ("DIO.1:0.IN"=w361:fxp<+,2,2>, "QE.CNTR"=→"ENC.C_0.CNTR":u32, "QE.STAT"=→"ENC.C_0.STAT":u8)  [unwired: 11 in]
    n139 = call "DIO 1-bit.vi"("DIR"=w367, "OUT"=w373, "DIO Refnum"=refnum<k21> "ConnectorC/DIO1") -> ("IN"=w360:bool)  [unwired: 8 in]
    n140 = call "DIO_PWM.vi"("DIO.OUT"=w372, "DIO.DIR"=w366, "PWM.CS"="PWM.C_0.CS", "PWM.CNFG"="PWM.C_0.CNFG", "PWM.CMP"="PWM.C_0.CMP", "PWM.MAX"="PWM.C_0.MAX", "DIO/PWM"=refnum<k21> "ConnectorC/DIO3", "SELECT"=w379) -> ("DIO.IN"=w359:bool, "PWM.CNTR"=→"PWM.C_0.CNTR":u16)  [unwired: 10 in]
    n141 = call "DIO_Encoder.vi"("DIO.1:0.OUT"=w371, "DIO.1:0.DIR"=w365, "QE.CNFG"="ENC.C_1.CNFG", "DIO.1/QE.B"=refnum<k21> "ConnectorC/DIO6", "SELECT"=w378, "DIO.0/QE.A"=refnum<k21> "ConnectorC/DIO4") -> ("DIO.1:0.IN"=w358:fxp<+,2,2>, "QE.CNTR"=→"ENC.C_1.CNTR":u32, "QE.STAT"=→"ENC.C_1.STAT":u8)  [unwired: 11 in]
    n142 = call "DIO 1-bit.vi"("DIR"=w364, "OUT"=w370, "DIO Refnum"=refnum<k21> "ConnectorC/DIO5") -> ("IN"=w357:bool)  [unwired: 8 in]
    n143 = call "DIO_PWM.vi"("DIO.OUT"=w369, "DIO.DIR"=w363, "PWM.CS"="PWM.C_1.CS", "PWM.CNFG"="PWM.C_1.CNFG", "PWM.CMP"="PWM.C_1.CMP", "PWM.MAX"="PWM.C_1.MAX", "DIO/PWM"=refnum<k21> "ConnectorC/DIO7", "SELECT"=w377) -> ("DIO.IN"=w356:bool, "PWM.CNTR"=→"PWM.C_1.CNTR":u16)  [unwired: 10 in]
    n144 = call "Join myDAQ DIO.vi"("IN 7"=w356, "IN 5"=w357, "IN 6, IN 4"=w358, "IN 2, IN 0"=w361, "IN 3"=w359, "IN 1"=w360) -> ("IN 7:0"=→"DIO.C_7:0.IN":u8)  [unwired: 4 in]
  }
  n145 = node-c288(w9) -> ()
